vi "get write location spread.vi"(11 "reader status":T1) -> (1 "2D indices":u32[](array[numeric]), 3 "3D write locations":u32[](array[numeric]))   [LabVIEW 2010]
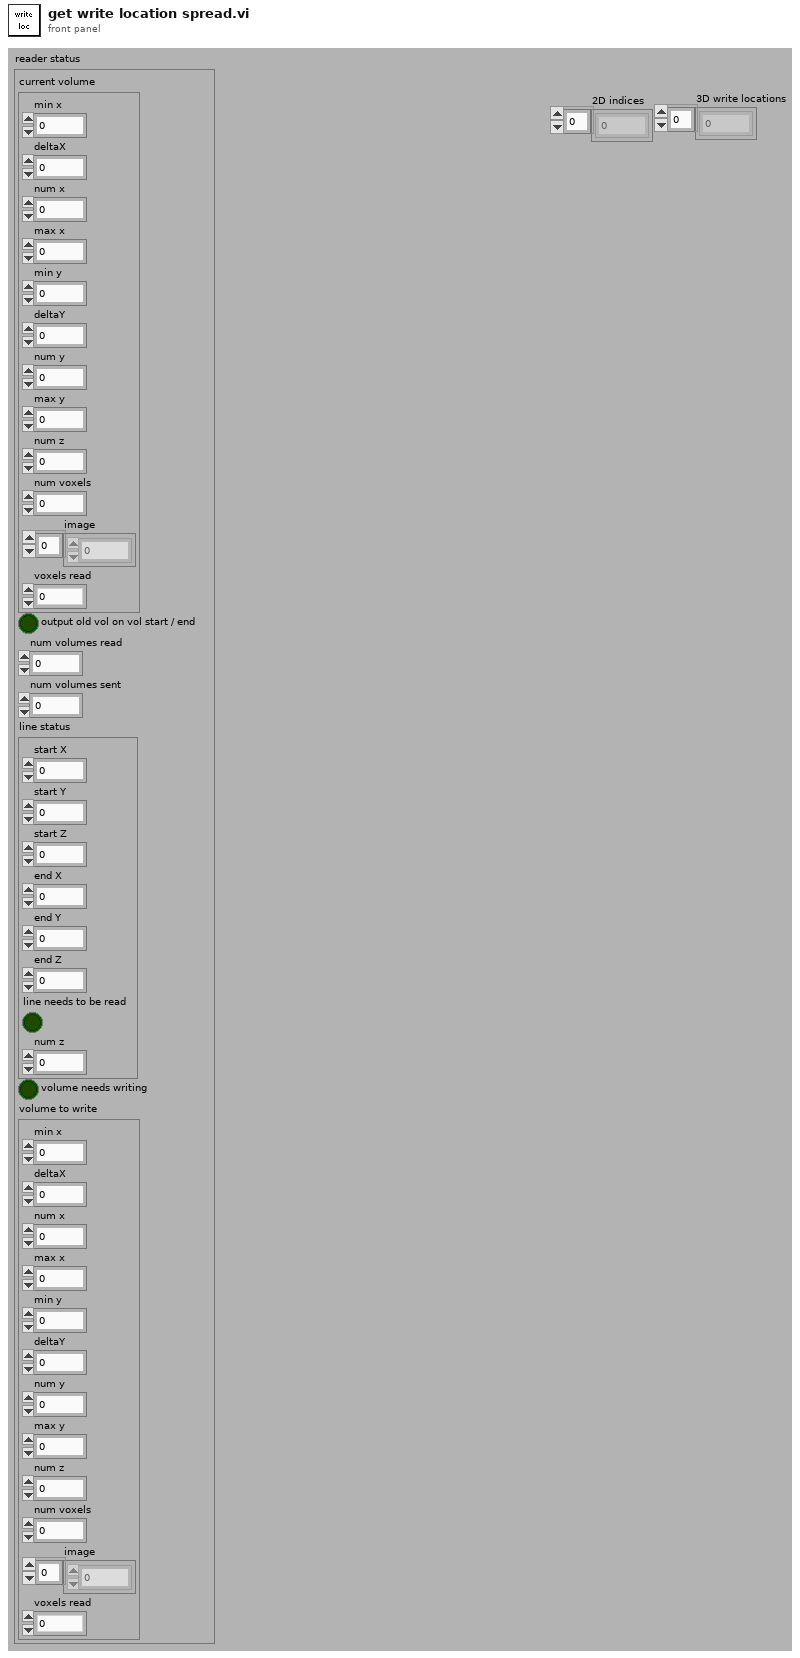
[diagram p1: front panel]
types:
  T1 = cluster{"current volume":cluster{"min x":i16, "deltaX":dbl, "num x":u32, "max x":i16, "min y":i16, "deltaY":dbl, "num y":u32, "max y":i16, "num z":u32, "num voxels":u32, "image":u32[], "voxels read":u32}, "output old vol on vol start / end":bool, "num volumes read":u32, "num volumes sent":u32, "line status":cluster{"start X":i16, "start Y":i16, "start Z":i16, "end X":i16, "end Y":i16, "end Z":i16, "line needs to be read":bool, "num z":u8}, "volume needs writing":bool, "volume to write":cluster{"min x":i16, "deltaX":dbl, "num x":u32, "max x":i16, "min y":i16, "deltaY":dbl, "num y":u32, "max y":i16, "num z":u32, "num voxels":u32, "image":u32[], "voxels read":u32}}
  T2 = cluster{"start X":i16, "start Y":i16, "start Z":i16, "end X":i16, "end Y":i16, "end Z":i16, "line needs to be read":bool, "num z":u8}
  T3 = cluster{"min x":i16, "deltaX":dbl, "num x":u32, "max x":i16, "min y":i16, "deltaY":dbl, "num y":u32, "max y":i16, "num z":u32, "num voxels":u32, "image":u32[], "voxels read":u32}
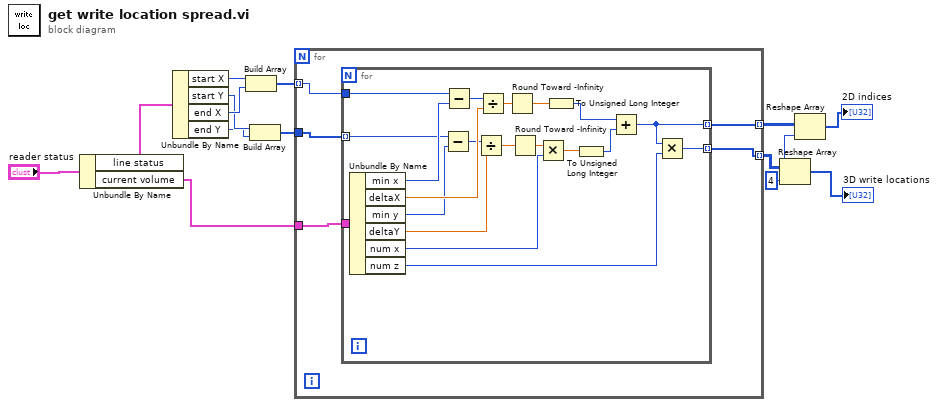
[diagram p0: block diagram]
diagram:
  w3 = 4 ("dimension size")
  n1 = Unbundle By Name("reader status") -> ("line status"=w12:T2, "current volume"=w13:T3)
  n2 = Unbundle By Name(w12) -> ("start X"=w11:i16, "start Y"=w9:i16, "end X"=w10:i16, "end Y"=w8:i16)
  n3 = Build Array(w11, w10) -> (w7:i16[])
  n4 = Build Array(w9, w8) -> (w6:i16[])
  n5 = for {
    tunnel: w13 -> [w19]
    tunnel: [w18] -> w4 mode=indexing
    tunnel: [w17] -> w5 mode=indexing
    tunnel: w7 -> [w16] mode=indexing
    tunnel: w6 -> [w15]
    n6 = for {
      tunnel: w19 -> [w39]
      tunnel: [w24] -> w18 mode=indexing
      tunnel: [w22] -> w17 mode=indexing
      tunnel: w16 -> [w21]
      tunnel: w15 -> [w20] mode=indexing
      n7 = Unbundle By Name(w39) -> ("min x"=w38:i16, "deltaX"=w36:dbl, "min y"=w34:i16, "deltaY"=w32:dbl, "num x"=w29:u32, "num z"=w23:u32)
      n8 = Subtract(x=w20, y=w34) -> (x-y=w33:i16)
      n9 = Subtract(x=w21, y=w38) -> (x-y=w37:i16)
      n10 = Divide(x=w33, y=w32) -> (x/y=w31:dbl)
      n11 = Divide(x=w37, y=w36) -> (x/y=w35:dbl)
      n12 = Round Toward -Infinity(1:w35) -> (0:w28:dbl)
      n13 = Round Toward -Infinity(1:w31) -> (0:w30:dbl)
      n14 = Multiply(x=w30, y=w29) -> (x*y=w27:dbl)
      n15 = To Unsigned Long Integer(number=w28) -> (unsigned 32bit integer=w26:u32)
      n16 = To Unsigned Long Integer(number=w27) -> (unsigned 32bit integer=w25:u32)
      n17 = Add(x=w26, y=w25) -> (x+y=w24:u32)
      n18 = Multiply(x=w24, y=w23) -> (x*y=w22:u32)
    }
  }
  n19 = Reshape Array(w5, w3) -> (→"3D write locations":u32[])
  n20 = Reshape Array(w4, w3) -> (→"2D indices":u32[])
